vi "Find slice locations from file.vi"() -> ()   [LabVIEW 2013, in "Tiff reader.lvlib"]
uses:
  Tiff reader.lvlib
panel:
  out "error out":errorcluster
  in  "error in (no error)":errorcluster
  in  "file path (use dialog)":path
  out "Slice start positions":u32[](array[numeric])
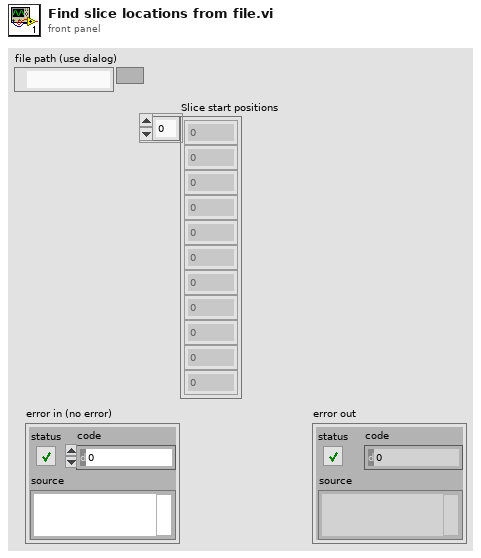
[diagram p1: front panel]
types:
  T1 = enum16{"open", "replace", "create", "open or create", "replace or create", "replace or create with confirmation"}
  T2 = typedef "Tiff reader.lvlib/IFD Entry.ctl" = cluster{"Tag":u16, "Type":T3, "Count":u32, "Val/Offs":u32, "Is Pointer?":bool, "Byte stream index":i32}
  T3 = typedef "Tiff reader.lvlib/FieldTypes.ctl" = enum16{"NULL", "U8", "ASCII7", "U16", "U32", "RATIONAL", "SByte(I8)", "Undef(8Bit)", "I16", "I32", "SRat(4B:4B)", "SGL(4Byte)", "DBL(8Byte)"}
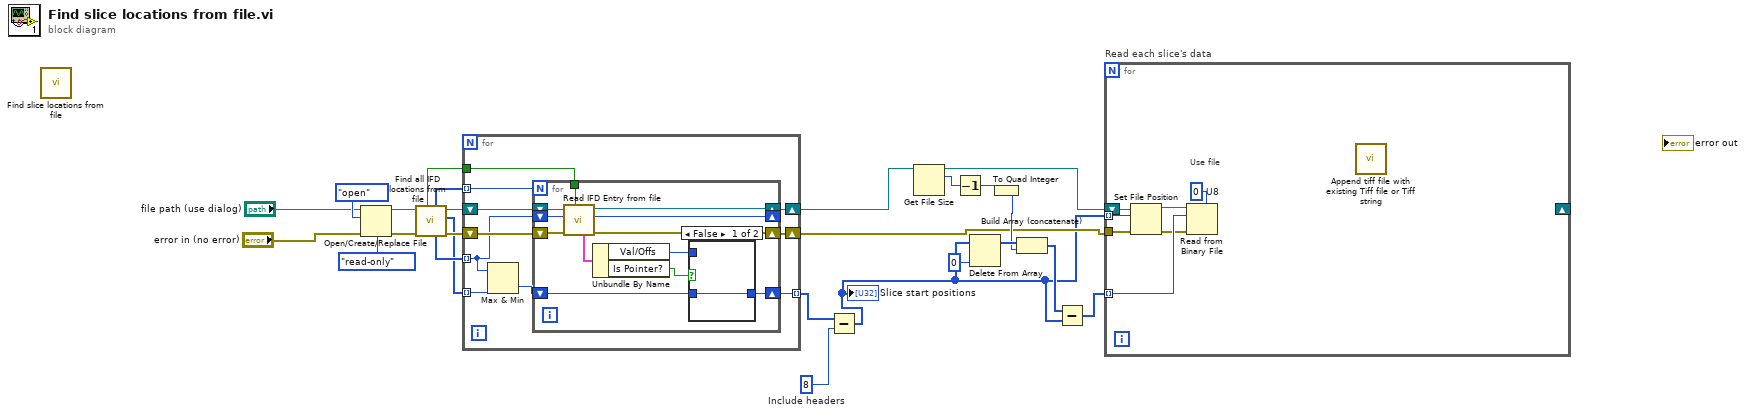
[diagram p0: block diagram]
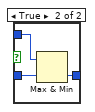
[diagram p2: hidden frame]
diagram:
  w1 = 8  # Include headers
  n1 = call "Find slice locations from file.vi"() -> ()  [unwired: 12 in]
  n2 = Open/Create/Replace File(file path (use dialog)="file path (use dialog)", error in="error in (no error)", operation (0:open)=T1."open", access (0:read/write)=enum16{"read/write", "read-only", "write-only"}."read-only") -> (refnum out=w23:refnum<file>, error out=w22:errorcluster)  [unwired: 3 out]
  n3 = call "Find all IFD locations from file.vi"("error in"=w22, "File"=w23) -> ("error out"=w21:errorcluster, "IFD locations"=w16:u32[], "File"=w17:refnum<file>, "1st tag locations"=w20:u32[], "# of tags in each IFD"=w18:u16[], "Litt/BigEnd"=w19:bool)  [unwired: 4 out]
  n4 = for {
    tunnel: w20 -> [w31] mode=indexing
    tunnel: w19 -> [w34]
    tunnel: w18 -> [w33] mode=indexing
    shift-right: [w27] -> w12
    shift-left: w17 -> [w32]
    tunnel: w16 -> [w30] mode=indexing
    tunnel: [w28] -> w3 mode=indexing
    shift-right: [w26] -> w4
    shift-left: w21 -> [w35]
    n5 = Max & Min(x=w31, y=w30) -> (min(x,y)=w29:u32)  [unwired: 1 out]
    n6 = for {
      N: w33 -> [_]
      shift-right: [w43] -> w27
      shift-left: w32 -> [w47]
      shift-right: [w44] -> _
      shift-left: w31 -> [w41]
      tunnel: w34 -> [w42]
      shift-right: [w45] -> w26
      shift-left: w35 -> [w46]
      shift-right: [w38] -> w28
      shift-left: w29 -> [w39]
      n7 = call "Read IFD Entry from file.vi"("Litt/BigEnd"=w42, "error in"=w46, "Tag location in"=w41, "File"=w47) -> ("error out"=w45:errorcluster, "Next Tag location Out\n(IN + 12)"=w44:i64, "File"=w43:refnum<file>, "Tag"=w40:T2)  [unwired: 1 in, 3 out]
      n8 = Unbundle By Name(w40) -> ("Val/Offs"=w37:u32, "Is Pointer?"=w36:bool)
      n9 = case shown="False" w36 {
        tunnel: w39 -> [w48 w51]
        tunnel: [w48 w50] -> w38
        tunnel: w37 -> [_ w49]
        frame False {
        }
        frame True {
          n10 = Max & Min(x=w49, y=w51) -> (min(x,y)=w50:u32)  [unwired: 1 out]
        }
      }
    }
  }
  n11 = Subtract(x=w3, y=w1) -> (x-y=w2:u32[])
  "Slice start positions" <- w2
  n12 = Get File Size(file=w12) -> (refnum out=w11:refnum<file>, size (in bytes)=w13:i64)  [unwired: 1 in, 1 out]
  n13 = Decrement(x=w13) -> (x-1=w8:i64)
  n14 = Delete From Array(array=w2, index=0) -> (array with subset deleted=w9:u32[])  [unwired: 1 in, 1 out]
  n15 = To Quad Integer(1:w8) -> (0:w7:i64)
  n16 = Build Array (concatenate)(w9, w7) -> (w6:i64[])
  n17 = Subtract(x=w6, y=w2) -> (x-y=w5:i64[])
  n18 = for "Read each slice's data" {
    tunnel: w2 -> [w56] mode=indexing
    tunnel: w5 -> [w54] mode=indexing
    shift-right: _ -> [_]
    shift-left: w11 -> [w57]
    tunnel: w4 -> [w52]
    w58 = u8 0  # U8
    # "Use file"
    n19 = Set File Position(offset (in bytes) (0)=w56, refnum=w57, error in=w52) -> (refnum out=w55:refnum<file>, error out=w53:errorcluster)  [unwired: 1 in]
    n20 = Read from Binary File(5:w58, 8:w53, 10:w54, 11:w55) -> ()  [unwired: 6 out]
    n21 = call "Append tiff file with existing Tiff file or Tiff string.vi"() -> ()  [unwired: 13 in, 3 out]
  }
